vi "XB.vi"   [LabVIEW 2020]
types:
  T1 = typedef "WPI_JoystickDevRef.ctl" = cluster{"Device":T2}
  T2 = typedef "WPI_JoystickDeviceEnum.ctl" = enum16{"USB 0", "USB 1", "USB 2", "USB 3", "USB 4", "USB 5"}
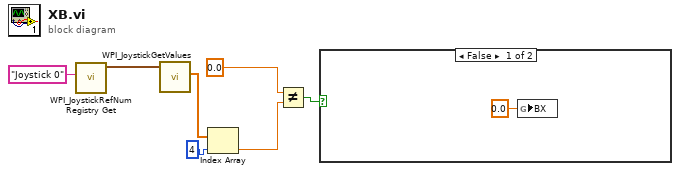
[diagram p0: block diagram]
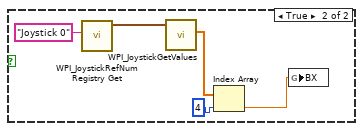
[diagram p2: hidden frame]
diagram:
  n1 = call <vilib>:"WPI_JoystickRefNum Registry Get.vi"("refnum name"="Joystick 0") -> ("JoystickDevRef"=w6:T1)  [unwired: 9 in, 1 out]
  n2 = call <vilib>:"WPI_JoystickGetValues.vi"("JoystickDevRef"=w6) -> ("Axes"=w5:dbl[])  [unwired: 6 in, 4 out]
  n3 = Index Array(array=w5, index=4) -> (element=w3:dbl)
  n4 = Not Equal?(x=0.0, y=w3) -> (x != y?=w1:bool)
  n5 = case shown="False" w1 {
    frame False {
      n6 = global write "XB.vi" "BX"(0.0 ("BX")) -> ()
    }
    frame True {
      n7 = call <vilib>:"WPI_JoystickRefNum Registry Get.vi"("refnum name"="Joystick 0") -> ("JoystickDevRef"=w12:T1)  [unwired: 9 in, 1 out]
      n8 = call <vilib>:"WPI_JoystickGetValues.vi"("JoystickDevRef"=w12) -> ("Axes"=w11:dbl[])  [unwired: 6 in, 4 out]
      n9 = Index Array(array=w11, index=4) -> (element=w9:dbl)
      n10 = global write "XB.vi" "BX"(w9) -> ()
    }
  }
